vi "PCO_GetRecordStopEvent.vi"(8 "error in (no error)":errorcluster {"code" format="%x"}, 11 "ph":u64) -> (0 "error out":errorcluster {"code" format="%x"}, 1 "wRecordStopEventMode":u16(ring) items=["OFF", "software", "extern"], 2 "ErrorMessage":i32 format="%x", 3 "ph out":u64, 5 "dwRecordStopDelayImages":u32)   [LabVIEW 2019, in "SDK.lvlib" / "RecordingControl.lvlib"]
doc: "<b>Description:</b>\nThis function returns the current record stop event mode and the number of images, which will be recorded after a recorder stop event is triggered.\nThe record stop event mode is only valid, if storage mode is [recorder] and recorder submode is [ring buffer].\n\n<b>Supported camera type:</b>\npco.1200, pco.dimax\n\n<b>Descriptor dependency:</b>\ndwGeneralCapsDESC1: RECORD_STOP"
uses:
  RecordingControl.lvlib
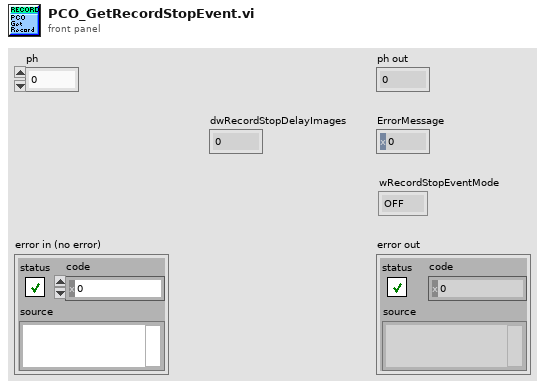
[diagram p1: front panel]
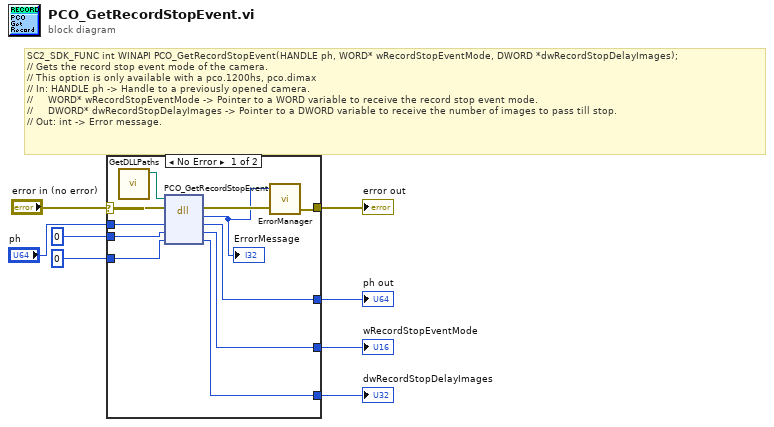
[diagram p0: block diagram]
diagram:
  # "SC2_SDK_FUNC int WINAPI PCO_GetRecordStopEvent(HANDLE ph, WORD* wRecordStopEventMode, DWORD *dwRecordStopDelayImages);\n// Gets the record stop event mode of the camera.\n// This option is only available with a pco.1200hs, pco.dimax\n// In: HANDLE ph -> Handle to a previously opened camera.\n//     WORD* wRecordStopEventMode -> Pointer to a WORD variable to receive the record stop event mode.\n//     DWORD* dwRecordStopDelayImages -> Pointer to a DWORD variable to receive the number of images to pass till stop.\n// Out: int -> Error message."
  n1 = case shown="No Error" "error in (no error)" {
    selector: "error in (no error)" -> [w13 w23]
    tunnel: "ph" -> [w19 w22]
    tunnel: [w18 w22] -> w7
    tunnel: u16 0 ("wRecordStopEventMode") -> [w17 w21]
    tunnel: [w16 w21] -> w5
    tunnel: u32 0 ("dwRecordStopDelayImages") -> [w15 w20]
    tunnel: [w14 w20] -> w3
    tunnel: [w11 w23] -> w2
    frame No Error {
      n2 = call "GetDLLPaths.vi"() -> ("SC2_Cam_Path"=w9:path)  [unwired: 8 in, 3 out]
      n3 = dll-call lib="?" fn="PCO_GetRecordStopEvent"(path in=w9, error in=w13, "ph"=w19, "wRecordStopEventMode"=w17, "dwRecordStopDelayImages"=w15) -> (error out=w12:errorcluster, "return type"=w10:i32, "ph"=w18:u64, "wRecordStopEventMode"=w16:u16, "dwRecordStopDelayImages"=w14:u32)  [unwired: 1 in, 1 out]
      "ErrorMessage" <- w10
      n4 = call "ErrorManager.vi"("error in (no error)"=w12, "error code"=w10) -> ("error out"=w11:errorcluster)  [unwired: 2 in, 1 out]
    }
    frame Error {
    }
  }
  "ph out" <- w7
  "wRecordStopEventMode" <- w5
  "dwRecordStopDelayImages" <- w3
  "error out" <- w2
